vi "Set New Position Values.vi"(9 "Data":u16, 10 "Came From Detect?":bool, 11 "State Data in":T1) -> (3 "State Data out":T1)   [LabVIEW 2015, in "Engine Simulation Toolkit.lvlib" / "Directional Speed.lvlib"]
uses:
  Directional Speed.lvlib
  State Data.ctl
  Settings.ctl
  State.ctl
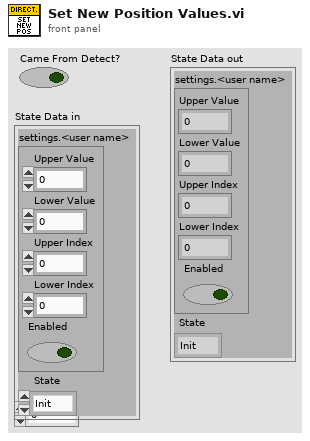
[diagram p1: front panel]
types:
  T1 = typedef "Engine Simulation Toolkit.lvlib/Directional Speed.lvlib/State Data.ctl" = cluster{"settings.<user name>":T2, "State":T3}
  T2 = typedef "Engine Simulation Toolkit.lvlib/Directional Speed.lvlib/Settings.ctl" = cluster{"Upper Value":u16, "Lower Value":u16, "Upper Index":fxp<+,10,10>, "Lower Index":fxp<+,10,10>, "Enabled":bool}
  T3 = typedef "Engine Simulation Toolkit.lvlib/Directional Speed.lvlib/State.ctl" = enum8{"Init", "Detect", "Positive Move td", "Negative Move td", "tf", "tr"}
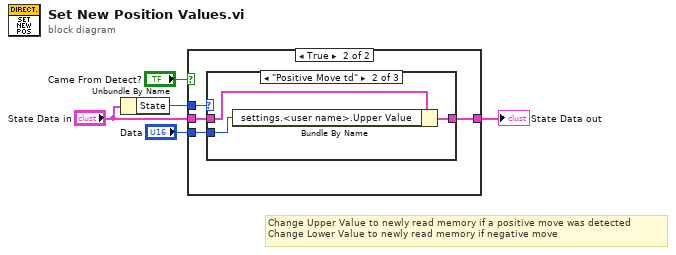
[diagram p0: block diagram]
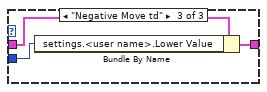
[diagram p4: hidden frame]
diagram:
  # "Change Upper Value to newly read memory if a positive move was detected\nChange Lower Value to newly read memory if negative move"
  n1 = Unbundle By Name("State Data in") -> ("State"=w2:T3)
  n2 = case shown="True" "Came From Detect?" {
    tunnel: w2 -> [_ w10]
    tunnel: "State Data in" -> [w6 w9]
    tunnel: "Data" -> [_ w8]
    tunnel: [w6 w7] -> w5
    frame False {
    }
    frame True {
      n3 = case shown="\"Positive Move td\"" w10 {
        tunnel: w9 -> [w11 w14 w17]
        tunnel: w8 -> [_ w13 w16]
        tunnel: [w11 w12 w15] -> w7
        frame Default {
        }
        frame "Positive Move td" {
          n4 = Bundle By Name(cluster=w14, "settings.<user name>.Upper Value"=w13) -> (w12:T1)
        }
        frame "Negative Move td" {
          n5 = Bundle By Name(cluster=w17, "settings.<user name>.Lower Value"=w16) -> (w15:T1)
        }
      }
    }
  }
  "State Data out" <- w5
